vi "dummy_out.vi"(5 "IN VARIANT":variant, 7 "ip":string, 9 "Name in":string) -> (10 "Operation Ok":bool)   [LabVIEW 2015]
uses:
  LI_states.ctl
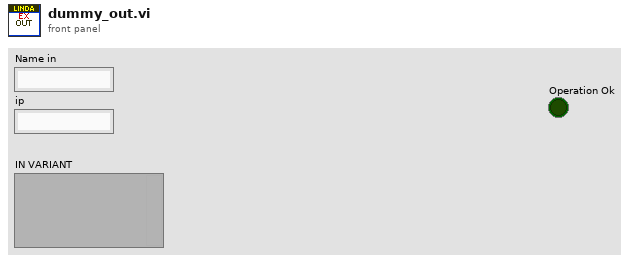
[diagram p1: front panel]
types:
  T1 = typedef "LI_states.ctl" = enum16{"Out", "In", "Rd", "Inp", "Rdp", "Init", "Cleanup", "RdAll"}
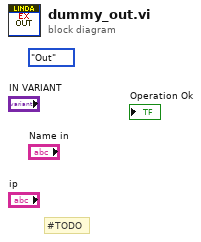
[diagram p0: block diagram]
diagram:
  (unwired) LI_states."Out" ("OP")
  # "#TODO"
